vi "Script - delete frame.vi"(8 "errorin":errorcluster, 9 "Structure Type":T1, 10 "Frame Index":u32, 11 "StructRef":refnum<vi>) -> (0 "error out":errorcluster)   [LabVIEW 2020]
uses:
  StructureTypes.ctl
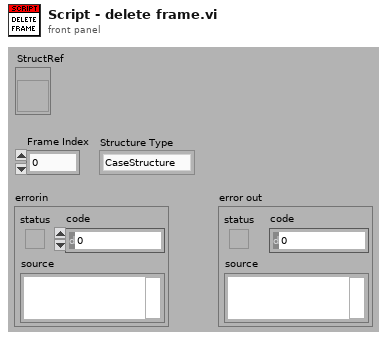
[diagram p1: front panel]
types:
  T1 = typedef "StructureTypes.ctl" = enum16{"CaseStructure", "EventStructure"}
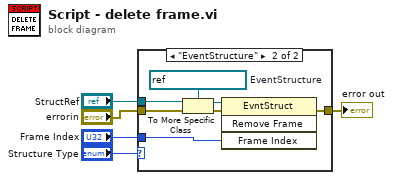
[diagram p0: block diagram]
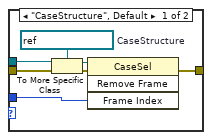
[diagram p2: hidden frame]
diagram:
  n1 = case shown="\"EventStructure\"" "Structure Type" {
    tunnel: "Frame Index" -> [w12 w19]
    tunnel: "StructRef" -> [w8 w15]
    tunnel: [w11 w18] -> w3
    tunnel: "errorin" -> [w9 w16]
    frame "CaseStructure", Default {
      w6 = refnum<vi> refnum  # CaseStructure
      n2 = To More Specific Class(target class=w6, reference=w8, error in=w9) -> (specific class reference=w7:refnum<vi>, error out=w10:errorcluster)
      n3 = invoke class="CaseSel" method="Remove Frame"(reference=w7, error in=w10, "Frame Index"=w12) -> (error out=w11:errorcluster)  [unwired: 1 in, 3 out]
    }
    frame "EventStructure" {
      w13 = refnum<vi> refnum  # EventStructure
      n4 = To More Specific Class(target class=w13, reference=w15, error in=w16) -> (specific class reference=w14:refnum<vi>, error out=w17:errorcluster)
      n5 = invoke class="EvntStruct" method="Remove Frame"(reference=w14, error in=w17, "Frame Index"=w19) -> (error out=w18:errorcluster)  [unwired: 1 in, 3 out]
    }
  }
  "error out" <- w3
